vi "WirteEDVR_Community.vi"(8 "error in":errorcluster, 11 "Edvr":T1) -> (0 "error out":errorcluster, 3 "NET":refnum<class "NET.lvclass">)   [LabVIEW 2020, in "OpenLvVision_OpenCv.lvlib" / "NET.lvclass"]
uses:
  NET.lvclass
  _LvHelpers/EdvrObject/EdvrObject.lvclass
  C:/Users/lukas/Downloads/OpenLvVision_OpenCv/SourceCode/LabView/OpenLvVision_OpenCv/_LvHelpers/EdvrObject/EdvrObject.lvclass
  C:/Users/lukas/Downloads/OpenLvVision_OpenCv/SourceCode/LabView/OpenLvVision_OpenCv/DNN/NET/NET.lvclass
  _LvHelpers/EdvrObject/TypeDef/Edvr.ctl
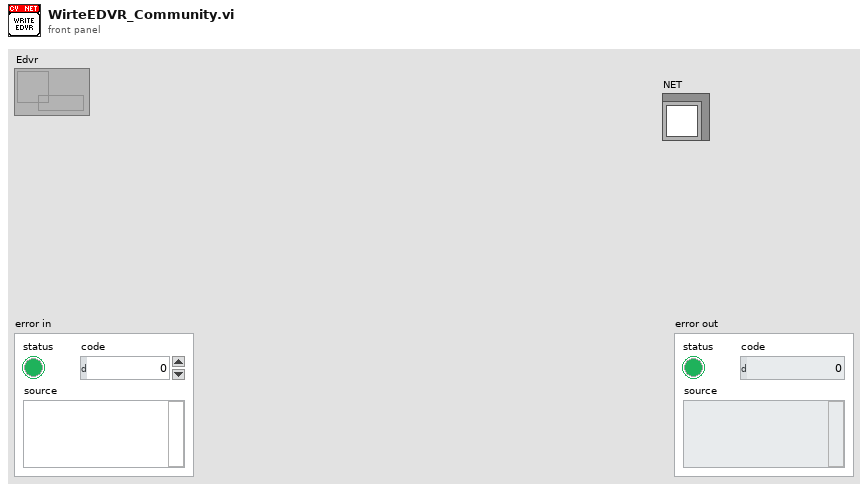
[diagram p1: front panel]
types:
  T1 = typedef "OpenLvVision_OpenCv.lvlib/EdvrObject.lvclass/Edvr.ctl" = refnum<data-value>
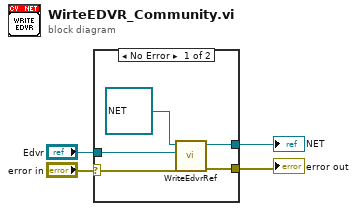
[diagram p0: block diagram]
diagram:
  n1 = case shown="No Error" "error in" {
    selector: "error in" -> [w9 w10]
    tunnel: "Edvr" -> [w7 _]
    tunnel: [w6 w10] -> w1
    tunnel: [w5 _] -> w2
    frame No Error {
      n2 = call "WriteEdvrRef.vi"("error in (no error)"=w9, "Edvr"=w7, "EdvrObject in"=refnum<class "NET.lvclass"> refnum ("NET")) -> ("error out"=w6:errorcluster, "EdvrObject out"=w5:refnum<class "NET.lvclass">)  [unwired: 7 in]
    }
    frame Error {
    }
  }
  "error out" <- w1
  "NET" <- w2
